vi "UpdateNotes.vi"(8 "error in (no error)":errorcluster, 11 "Experiment in":refnum<class "Experiment.lvclass">) -> (0 "error out":errorcluster, 3 "Experiment out":refnum<class "Experiment.lvclass">)   [LabVIEW 2014, in "Experiment.lvclass"]
uses:
  Experiment.lvclass
  Experiment.lvclass/Experiment.ctl
  Database/Database.lvclass
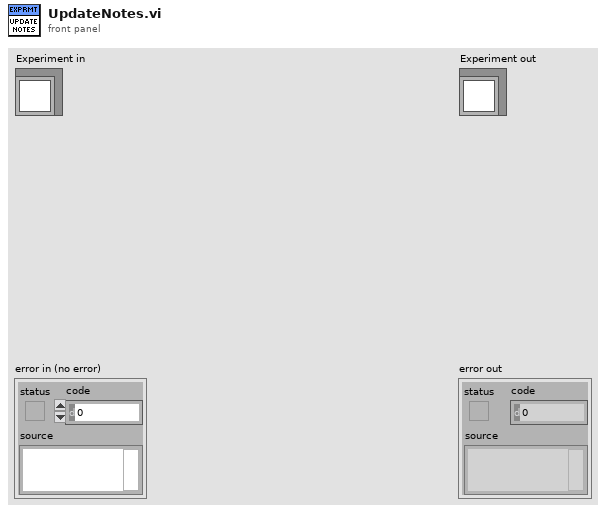
[diagram p1: front panel]
types:
  T1 = cluster{"session":dbl, "animal_id":dbl, "scan_idx":dbl}
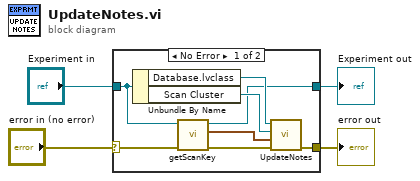
[diagram p0: block diagram]
diagram:
  n1 = case shown="No Error" "error in (no error)" {
    selector: "error in (no error)" -> [w7 w14]
    tunnel: [w5 w14] -> w3
    tunnel: [w8 w13] -> w1
    tunnel: "Experiment in" -> [w9 w13]
    frame No Error {
      n2 = Unbundle By Name(w9) -> ("Database.lvclass"=w12:refnum<class "Database.lvclass">, "Scan Cluster"=w11:refnum<vi>)
      n3 = call-dynamic "getScanKey.vi"("error in (no error)"=w7, "Experiment in"=w9) -> ("error out"=w6:errorcluster, "Scan Key"=w10:T1, "Experiment out"=w8:refnum<class "Experiment.lvclass">)  [unwired: 7 in]
      n4 = call-dynamic "UpdateNotes.vi"("error in (no error)"=w6, "Scan Key"=w10, "reference"=w11, "Database in"=w12) -> ("error out"=w5:errorcluster)  [unwired: 6 in, 1 out]
    }
    frame Error {
    }
  }
  "error out" <- w3
  "Experiment out" <- w1
